vi "Read Camera Name.vi"(8 "error in (no error)":errorcluster, 10 "IMAQdx Data":T1 {"SerialNumberHigh" format="%x"; "SerialNumberLow" format="%x"}, 11 "Config File Directory":path) -> (0 "error out":errorcluster, 2 "Camera Name":string)   [LabVIEW 2011]
uses:
  <vilib>/Utility/config.llb/Read Key (String).vi
  <vilib>/Utility/config.llb/NI_LVConfig.lvlib
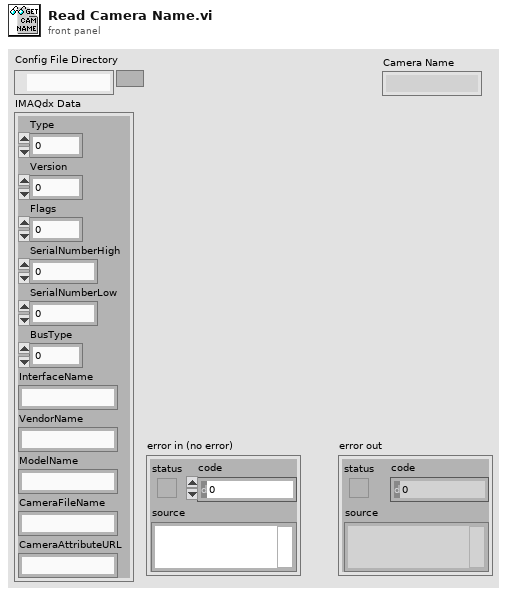
[diagram p1: front panel]
types:
  T1 = cluster{"Type":u32, "Version":u32, "Flags":u32, "SerialNumberHigh":u32, "SerialNumberLow":u32, "BusType":u32, "InterfaceName":string, "VendorName":string, "ModelName":string, "CameraFileName":string, "CameraAttributeURL":string}
  T2 = typedef "NI_LVConfig.lvlib/Config Data RefNum.ctl" = refnum<k1>
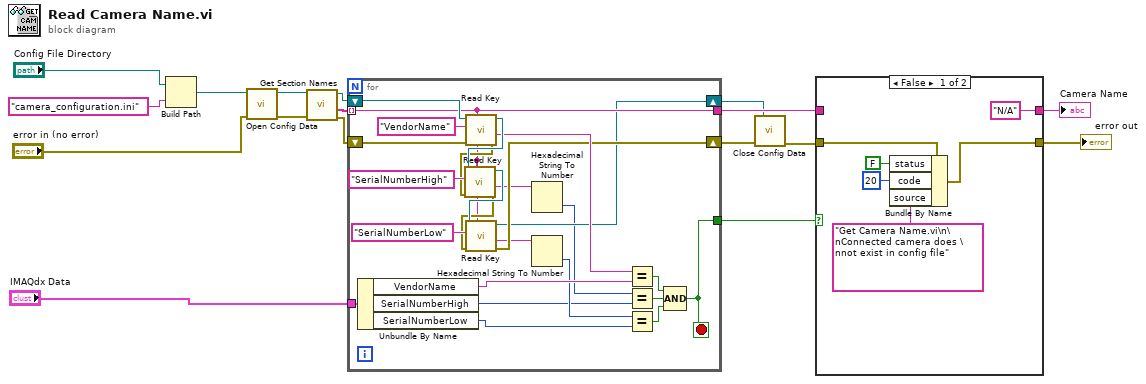
[diagram p0: block diagram]
diagram:
  n1 = Build Path(base path="Config File Directory", name or relative path="camera_configuration.ini") -> (appended path=w15:path)
  n2 = call <vilib>:"Open Config Data.vi"("error in (no error)"="error in (no error)", "configuration file path"=w15) -> ("error out"=w13:errorcluster, "refnum"=w12:T2)  [unwired: 7 in, 1 out]
  n3 = call <vilib>:"Get Section Names.vi"("error in (no error)"=w13, "refnum"=w12) -> ("error out"=w8:errorcluster, "section names"=w11:string[], "refnum out"=w9:T2)  [unwired: 7 in]
  n4 = for {
    tunnel: w11 -> [w27] mode=indexing
    tunnel: "IMAQdx Data" -> [w35]
    tunnel: [w25] -> w7
    tunnel: [w27] -> w6
    shift-right: [w26] -> w3
    shift-left: w8 -> [w30]
    shift-right: [w24] -> w4
    shift-left: w9 -> [w39]
    stop <- w25 stop-if-true
    n5 = Unbundle By Name(w35) -> ("VendorName"=w34:string, "SerialNumberHigh"=w18:u32, "SerialNumberLow"=w21:u32)
    n6 = call-poly <vilib>:"Read Key.vi"("section"=w27, "error in (no error)"=w30, "key"="VendorName", "refnum"=w39) -> ("error out"=w29:errorcluster, "value"=w36:string, "refnum out"=w38:T2)  [unwired: 4 in, 1 out]
    n7 = call-poly <vilib>:"Read Key.vi"("section"=w27, "error in (no error)"=w29, "key"="SerialNumberHigh", "refnum"=w38) -> ("error out"=w28:errorcluster, "value"=w23:string, "refnum out"=w37:T2)  [unwired: 4 in, 1 out]
    n8 = call-poly <vilib>:"Read Key.vi"("section"=w27, "error in (no error)"=w28, "key"="SerialNumberLow", "refnum"=w37) -> ("error out"=w26:errorcluster, "value"=w22:string, "refnum out"=w24:T2)  [unwired: 4 in, 1 out]
    n9 = Hexadecimal String To Number(string=w23) -> (number=w19:u32)  [unwired: 2 in, 1 out]
    n10 = Hexadecimal String To Number(string=w22) -> (number=w20:u32)  [unwired: 2 in, 1 out]
    n11 = Equal?(x=w36, y=w34) -> (x = y?=w33:bool)
    n12 = Equal?(x=w19, y=w18) -> (x = y?=w32:bool)
    n13 = Equal?(x=w20, y=w21) -> (x = y?=w31:bool)
    n14 = Compound Arithmetic op=AND(w33, w32, w31) -> (w25:bool)
  }
  n15 = call <vilib>:"Close Config Data.vi"("error in (no error)"=w3, "refnum"=w4) -> ("error out"=w2:errorcluster)  [unwired: 8 in, 1 out]
  n16 = case shown="False" w7 {
    tunnel: w6 -> [_ w50]
    tunnel: ["N/A" ("String") w50] -> w1
    tunnel: [w46 w49] -> w5
    tunnel: w2 -> [w47 w49]
    frame False {
      n17 = Bundle By Name(cluster=w47, "status"=FALSE, "code"=20, "source"="Get Camera Name.vi\n\nConnected camera does \nnot exist in config file") -> (w46:errorcluster)
    }
    frame True {
    }
  }
  "error out" <- w5
  "Camera Name" <- w1
